vi "Cal Standard Default Directory.vi"() -> (0 "Path out":path)   [LabVIEW 2023, in "RFFixtureCharact.Instruments.lvlib" / "Cal Standard Factory.lvclass"]
uses:
  Cal Standard Factory.lvclass
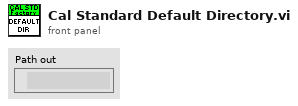
[diagram p1: front panel]
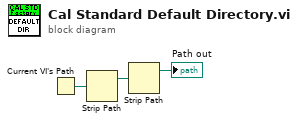
[diagram p0: block diagram]
diagram:
  n1 = Current VI's Path() -> (path=w3:path)
  n2 = Strip Path(path=w3) -> (stripped path=w2:path)  [unwired: 1 out]
  n3 = Strip Path(path=w2) -> (stripped path=→"Path out":path)  [unwired: 1 out]
